vi "Global 1.vi"() -> ()   [LabVIEW 2020]
panel:
  out "HAND":string="follow"
  out "Ch_sel":string="Index_U"
  out "Repeat_train":string="Index_U"
  out "Opt_met":string="Index_U"
  out "Rem_meth":string="Index_U"
  out "Max_p":string="Index_U"
  out "Prop":string="Index_U"
  out "FIXATION_PERIOD":string
  out "Test Protocol Iteration":dbl
  out "End Of Trial":bool
  out "BLOCKS_PER_DAY":string
  out "TRIALS_PER_BLOCK":string
  out "EEG_STREAM_CH8":string
  out "EEG_STREAM_CH7":string
  out "EEG_STREAM_CH6":string
  out "EEG_STREAM_CH5":string
  out "EEG_STREAM_CH4":string
  out "EEG_STREAM_CH3":string
  out "CHANNEL_SELECT_DEBUG":string="follow"
  out "MOVE":bool
  out "Rest":bool
  out "Movement Predicted":bool
  out "Imagine Movement":bool
  out "Fixate":bool
  out "CONGRATS_LEVEL":string="6"
  out "SYSTEM_STAGE":string="pacman"
  out "PROGRESS":string
  out "SVM_MODELS":string
  out "VI_RUNNING":string="0"
  out "TRIAL_NUMBER":string
  out "TASK":string="tracking"
  out "TARGET":string="100"
  out "HOME":string="0"
  out "TARGETS_ARRAY":string="0.01,0.9,0.3,0.78,0.46,0.83,0.42,0.88,0.38,0.96,0.33,0.91,0.51,0.1,0.88,0.42,0.98,0.54,0,0.87,0.22,0.99,0.33,0.82,0.44,0.07,0.86,0.18,0.81,0.25,0.82,0.21,0.6,0.14,0.46,0.89,0.07,0.95,0.49,0.07,0.44,0.75,0.19,0.74,0.11,0.56,0.05,0.66,0.21,0.64,0.96,0.19,0.8,0.42,0.04,0.58,0.92,0.02,0.57,0.93,0.29,0.9,0.29,0.77,0.13,0.5,0.08,0.68,0,0.51,0.88,0.13,0.66,0.09,0.65,0.31,0.99,0.25,0.96,0.53,0.91,0.24,0.6,0.2,0.88,0.16,0.91,0.18,0.69,0.16,0.49,0.04,0.43,0,0.88,0.36,0.8,0.19,0.63,0.1"
  out "PROCEDURE":string
  out "END_STAGE":string
  out "EOG_IMPEDANCES":string
  out "EEG_IMPEDANCES":string
  out "THERAPY_STAGE":string="move"
  out "DATE":string="07212021-16:55:25"
  out "SVM_TRAINING_PROGRESS":string="0"
  out "REDUCE_HEAD_MOVEMENT":bool
  out "LEVEL":string="medium"
  out "MODE":string="follow"
  out "VI_STREAM":string="19;9;9"
  out "EMERGENCY_STOP":string
  out "PAGE":string="Index_U"
  out "SURVEY":string
  out "EEG_STREAM_CH2":string
  out "POSITION":string="28"
  out "EEG_STREAM_CH1":string="19;9;9"
  # "Variables To LV :"
  # "Variables From LV :"
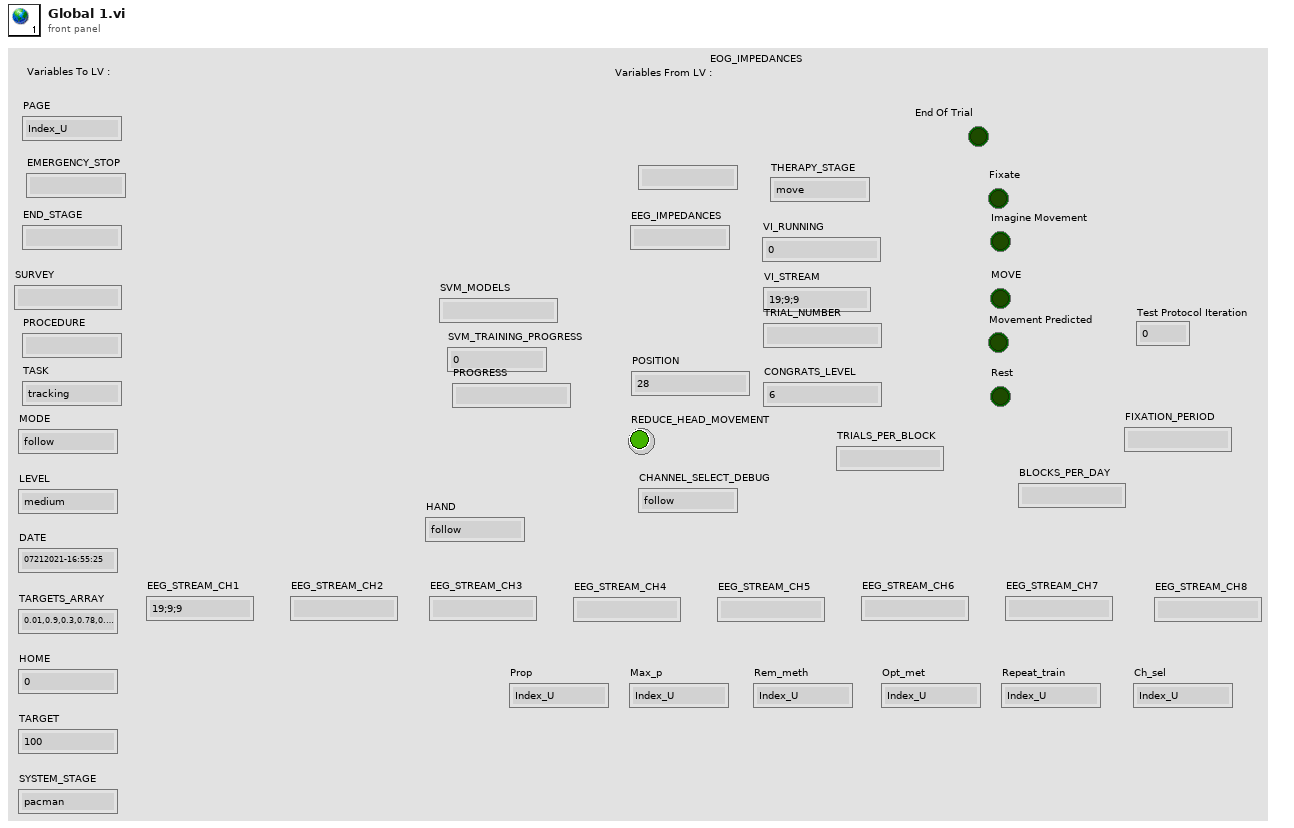
[diagram p1: front panel]
diagram:
